vi "Config Spark Max SLOT Close Loop HW Get Set.vi"(4 "PIDF Slot (0)":i32, 6 "Get(f) Set(t)":bool, 7 "SparkMax Slot CL":T1={"Gains"={"P"=0.1, "I"=0.0, "D"=0.0, "F"=0.0}, "I Zone"=1.0, "Peak Out -1 0 1"={"High"=0.0, "Low"=0.0}, "Max I Accu"=0.0} {"Gains"."F" format="%#.8f"; "Gains"."D" format="%#.8f"; "Gains"."I" format="%#.8f"; "Gains"."P" format="%#.8f"; "Peak Out -1 0 1"."Low" format="%#.8f"; "Peak Out -1 0 1"."High" format="%#.8f"}, 8 "Error":errorcluster, 11 "Drive Refs":T4) -> (0 "Error Out":errorcluster, 3 "Drive Refs Out":T4, 5 "SparkMax Slot CL Out":T1={"Gains"={"P"=0.1, "I"=0.0, "D"=0.0, "F"=0.0}, "I Zone"=1.0, "Peak Out -1 0 1"={"High"=0.0, "Low"=0.0}, "Max I Accu"=0.0} {"Gains"."F" format="%#.8f"; "Gains"."D" format="%#.8f"; "Gains"."I" format="%#.8f"; "Gains"."P" format="%#.8f"; "Peak Out -1 0 1"."Low" format="%#.8f"; "Peak Out -1 0 1"."High" format="%#.8f"})   [LabVIEW 2023, in "2024 AdvSwerve_ACT.lvlib"]
uses:
  2024 AdvSwerve_ACT.lvlib
  <vilib>/Rock Robotics/WPI/MotorControl/WPI_MotorControlDeviceRef.ctl
  <vilib>/Rock Robotics/WPI/MotorControl/WPI_MotorControlType.ctl
  <vilib>/Rock Robotics/SystemInterfaces/DIO/FPGA_DIOPWMChannel.ctl
  <vilib>/Rock Robotics/WPI/PWM/WPI_PWMDeadband.ctl
  <vilib>/Rock Robotics/SystemInterfaces/DIO/FPGA_DIOChannel.ctl
  Shared Code/TypeDefs/Cluster_Spark MAX Config_SLOT PID Config.ctl
  Shared Code/TypeDefs/Cluster_PID Gains.ctl
  Shared Code/TypeDefs/Cluster_High-Low.ctl
  Shared Code/TypeDefs/Cluster_SRX SLOT PID Config.ctl
  <vilib>/Utility/error.llb/Trim Whitespace One-Sided.vi
  <vilib>/Utility/Data Type/NI_Data Type.lvlib
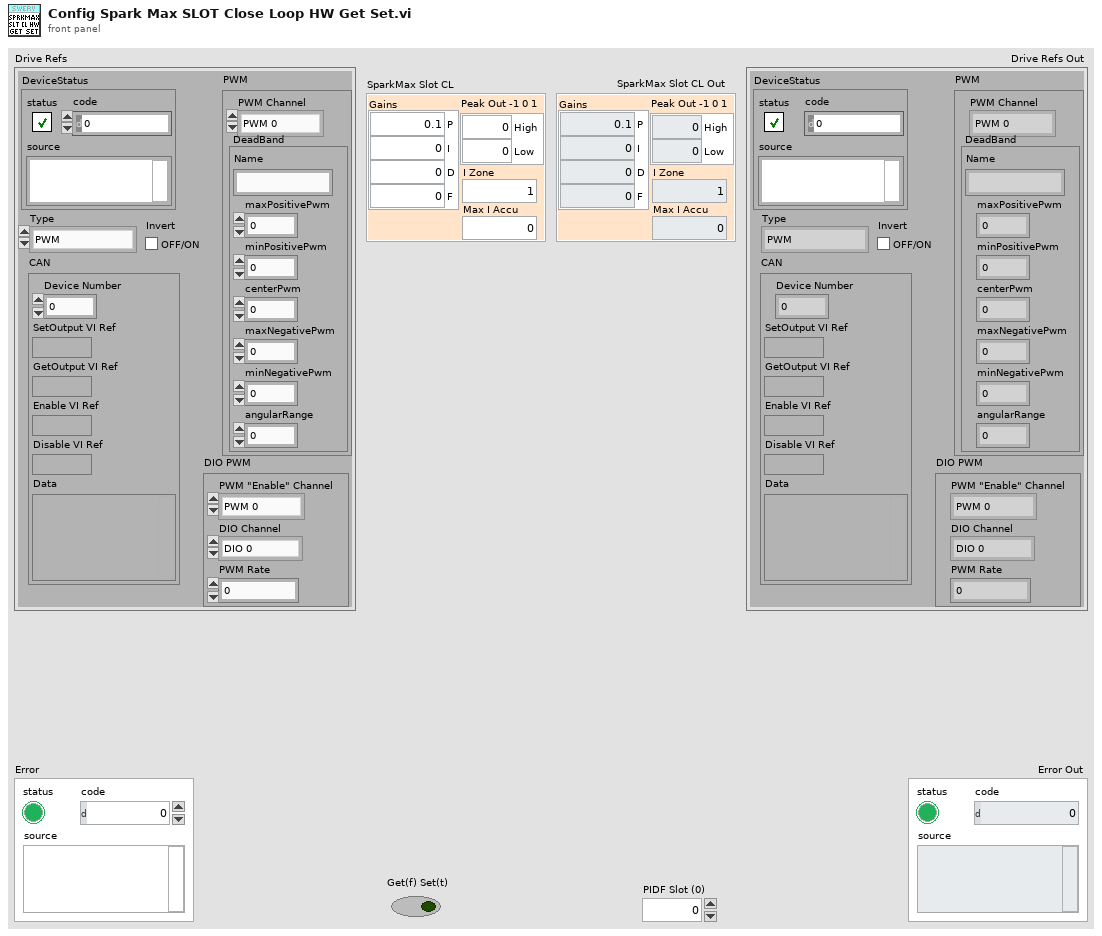
[diagram p1: front panel]
types:
  T1 = typedef "Cluster_Spark MAX Config_SLOT PID Config.ctl" = cluster{"Gains":T2, "I Zone":dbl, "Peak Out -1 0 1":T3, "Max I Accu":dbl}
  T2 = typedef "Cluster_PID Gains.ctl" = cluster{"P":dbl, "I":dbl, "D":dbl, "F":dbl}
  T3 = typedef "Cluster_High-Low.ctl" = cluster{"High":dbl, "Low":dbl}
  T4 = typedef "WPI_MotorControlDeviceRef.ctl" = cluster{"DeviceStatus":errorcluster, "Type":T5, "PWM":cluster{"PWM Channel":T6, "DeadBand":T7}, "CAN":cluster{"Device Number":u8, "SetOutput VI Ref":variant, "GetOutput VI Ref":variant, "Enable VI Ref":variant, "Disable VI Ref":variant, "Data":variant}, "Invert":bool, "DIO PWM":cluster{"PWM \"Enable\" Channel":T6, "DIOChannel":T8, "PWM Rate":dbl}}
  T5 = typedef "WPI_MotorControlType.ctl" = enum16{"PWM", "CAN", "DIO PWM"}
  T6 = typedef "FPGA_DIOPWMChannel.ctl" = enum8{"PWM 0", "PWM 1", "PWM 2", "PWM 3", "PWM 4", "PWM 5", "PWM 6", "PWM 7", "PWM 8", "PWM 9", "PWM MXP 0", "PWM MXP 1", "PWM MXP 2", "PWM MXP 3", "PWM MXP 4", "PWM MXP 5", "PWM MXP 6", "PWM MXP 7", "PWM MXP 8", "PWM MXP 9", "Invalid"}
  T7 = typedef "WPI_PWMDeadband.ctl" = cluster{"Name":string, "maxPositivePwm":i32, "minPositivePwm":i32, "centerPwm":i32, "maxNegativePwm":i32, "minNegativePwm":i32, "angularRange":u16}
  T8 = typedef "FPGA_DIOChannel.ctl" = enum8{"DIO 0", "DIO 1", "DIO 2", "DIO 3", "DIO 4", "DIO 5", "DIO 6", "DIO 7", "DIO 8", "DIO 9", "DIO MXP 0", "DIO MXP 1", "DIO MXP 2", "DIO MXP 3", "DIO MXP 4", "DIO MXP 5", "DIO MXP 6", "DIO MXP 7", "DIO MXP 8", "DIO MXP 9", "DIO MXP 10", "DIO MXP 11", "DIO MXP 12", "DIO MXP 13", "DIO MXP 14", "DIO MXP 15", "SPI Port CS1", "SPI Port CS2", "SPI Port CS3", "SPI Port MISO", "SPI Port MOSI", "Invalid"}
  T9 = typedef "Cluster_SRX SLOT PID Config.ctl" = cluster{"Gains":T2, "Error Allowed":dbl, "I Zone":dbl, "Peak Out 0-1":dbl, "Max I Accu":dbl}
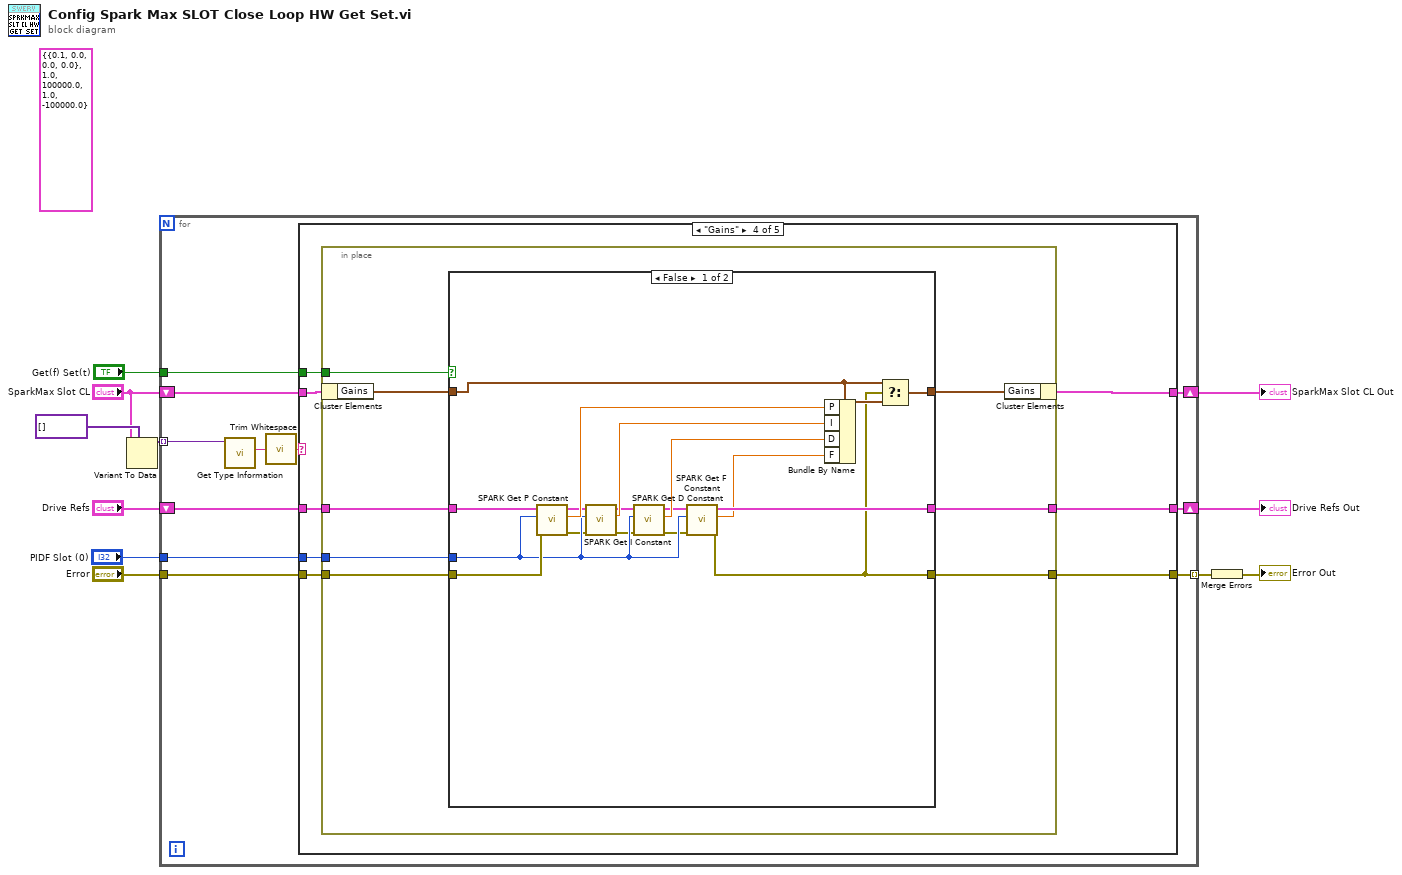
[diagram p0: block diagram]
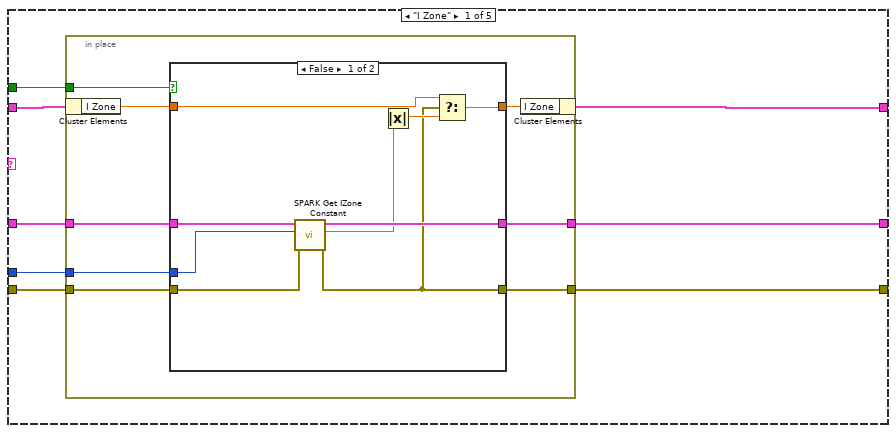
[diagram p2: hidden frame]
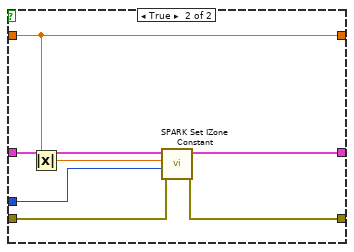
[diagram p3: hidden frame]
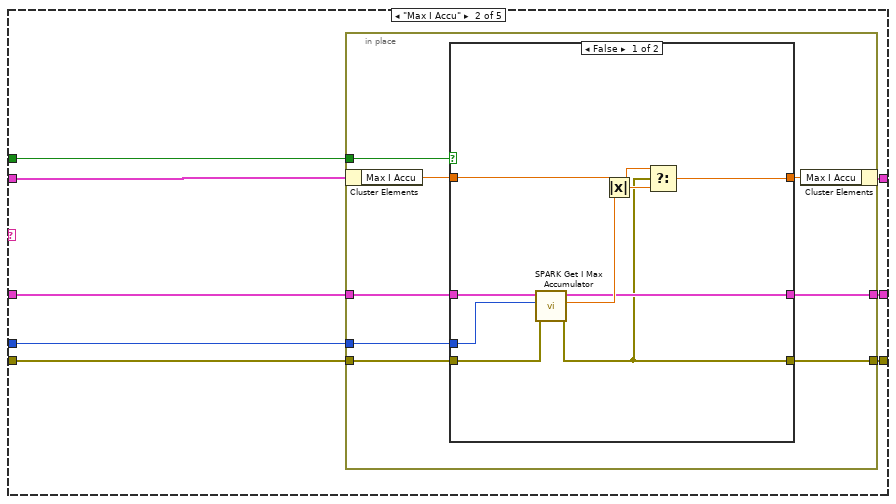
[diagram p4: hidden frame]
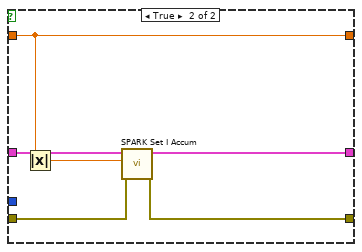
[diagram p5: hidden frame]
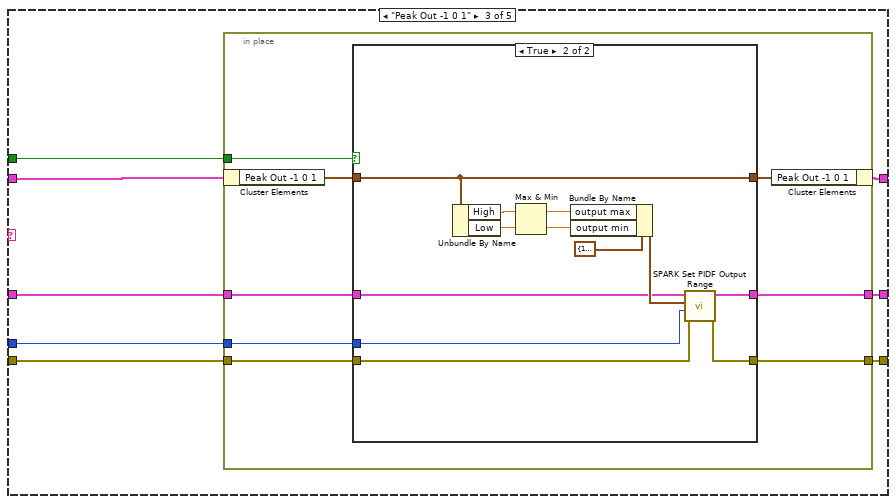
[diagram p6: hidden frame]
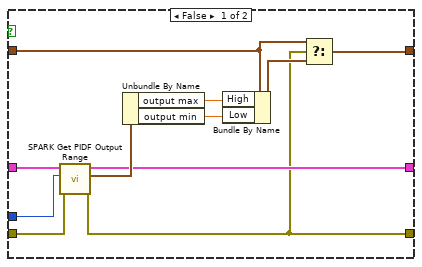
[diagram p7: hidden frame]
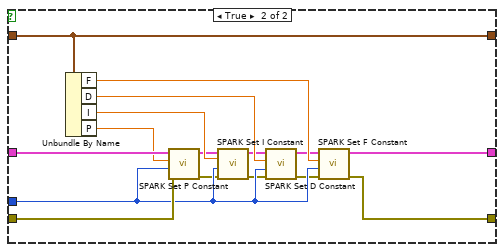
[diagram p8: hidden frame]
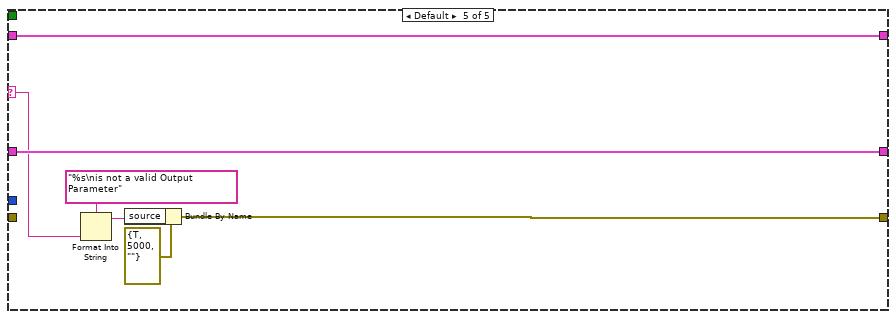
[diagram p9: hidden frame]
diagram:
  (unwired) T9 {"Gains"={"P"=0.1, "I"=0.0, "D"=0.0, "F"=0.0}, "Error Allowed"=1.0, "I Zone"=100000.0, "Peak Out 0-1"=1.0, "Max I Accu"=-100000.0} ("SparkMax Output")
  n1 = Variant To Data(type=variant[] [], Variant="SparkMax Slot CL") -> (data=w6:variant[])  [unwired: 1 in, 1 out]
  n2 = for {
    shift-right: [w13] -> w11
    shift-left: "SparkMax Slot CL" -> [w19]
    shift-right: [w14] -> w9
    shift-left: "Drive Refs" -> [w18]
    tunnel: "Get(f) Set(t)" -> [w17]
    tunnel: w6 -> [w21] mode=indexing
    tunnel: "Error" -> [w16]
    tunnel: [w15] -> w3 mode=indexing
    tunnel: "PIDF Slot (0)" -> [w12]
    n3 = call <vilib>:"Get Type Information.vi"("variant"=w21) -> ("name"=w22:string)  [unwired: 6 in, 4 out]
    n4 = call <vilib>:"Trim Whitespace.vi"("string"=w22) -> ("trimmed string"=w20:string)  [unwired: 1 in]
    n5 = case shown="\"Gains\"" w20 {
      selector: w20 -> [_ _ _ _ w179]
      tunnel: w19 -> [w30 w62 w93 w132 w181]
      tunnel: w18 -> [w26 w58 w89 w128 w180]
      tunnel: w17 -> [w29 w61 w92 w131 _]
      tunnel: w16 -> [w28 w60 w91 w130 _]
      tunnel: [w27 w59 w90 w129 w177] -> w15
      tunnel: [w25 w57 w88 w127 w180] -> w14
      tunnel: [w24 w56 w87 w126 w181] -> w13
      tunnel: w12 -> [w23 w55 w86 w125 _]
      frame "I Zone" {
        n6 = in-place {
          in-place-border: w29 -> [w38]
          in-place-border: w28 -> [w36]
          in-place-border: [w35] -> w27
          in-place-border: w26 -> [w34]
          in-place-border: [w33] -> w25
          in-place-border: w23 -> [w31]
          n7 = in-place-cluster #1(w30) -> ("I Zone"=w37:dbl)
          n8 = case shown="False" w38 {
            tunnel: w37 -> [w46 w54]
            tunnel: w36 -> [w40 w49]
            tunnel: [w39 w48] -> w35
            tunnel: w34 -> [w43 w53]
            tunnel: [w42 w52] -> w33
            tunnel: [w47 w54] -> w32
            tunnel: w31 -> [w44 w50]
            frame False {
              n9 = call <vilib>:"SPARK Get IZone Constant.vi"("error in (no error)"=w40, "PIDF Slot (0)"=w44, "MotorControlDeviceRef in"=w43) -> ("error out"=w39:errorcluster, "IZone"=w41:dbl, "MotorControlDeviceRef out"=w42:T4)  [unwired: 6 in]
              n10 = Absolute Value(x=w41) -> (abs(x)=w45:dbl)
              n11 = Select(t=w46, s=w39, f=w45) -> (s? t:f=w47:dbl)
            }
            frame True {
              n12 = Absolute Value(x=w54) -> (abs(x)=w51:dbl)
              n13 = call <vilib>:"SPARK Set IZone Constant.vi"("error in"=w49, "PIDF Slot"=w50, "IZone"=w51, "MotorControlDeviceRef"=w53) -> ("error out"=w48:errorcluster, "MotorControlDeviceRef"=w52:T4)  [unwired: 6 in]
            }
          }
          n14 = in-place-cluster #1("I Zone"=w32) -> (w24:T1)
        }
      }
      frame "Max I Accu" {
        n15 = in-place {
          in-place-border: w61 -> [w70]
          in-place-border: w60 -> [w68]
          in-place-border: [w67] -> w59
          in-place-border: w58 -> [w66]
          in-place-border: [w65] -> w57
          in-place-border: w55 -> [w63]
          n16 = in-place-cluster #2(w62) -> ("Max I Accu"=w69:dbl)
          n17 = case shown="False" w70 {
            tunnel: w69 -> [w78 w85]
            tunnel: w68 -> [w72 w81]
            tunnel: [w71 w80] -> w67
            tunnel: w66 -> [w74 w84]
            tunnel: [w75 w83] -> w65
            tunnel: [w79 w85] -> w64
            tunnel: w63 -> [w73 _]
            frame False {
              n18 = call <vilib>:"SPARK Get I Max Accumulator.vi"("error in (no error)"=w72, "PIDF Slot (0)"=w73, "MotorControlDeviceRef in"=w74) -> ("error out"=w71:errorcluster, "Max Accumulator"=w76:dbl, "MotorControlDeviceRef out"=w75:T4)  [unwired: 6 in]
              n19 = Absolute Value(x=w76) -> (abs(x)=w77:dbl)
              n20 = Select(t=w78, s=w71, f=w77) -> (s? t:f=w79:dbl)
            }
            frame True {
              n21 = Absolute Value(x=w85) -> (abs(x)=w82:dbl)
              n22 = call <vilib>:"SPARK Set I Accum.vi"("error in"=w81, "I Accum"=w82, "MotorControlDeviceRef"=w84) -> ("error out"=w80:errorcluster, "MotorControlDeviceRef"=w83:T4)  [unwired: 7 in]
            }
          }
          n23 = in-place-cluster #2("Max I Accu"=w64) -> (w56:T1)
        }
      }
      frame "Peak Out -1 0 1" {
        n24 = in-place {
          in-place-border: w92 -> [w101]
          in-place-border: w91 -> [w99]
          in-place-border: [w98] -> w90
          in-place-border: w89 -> [w97]
          in-place-border: [w96] -> w88
          in-place-border: w86 -> [w94]
          n25 = in-place-cluster #3(w93) -> ("Peak Out -1 0 1"=w100:T3)
          n26 = case shown="True" w101 {
            tunnel: w100 -> [w111 w123]
            tunnel: w99 -> [w103 w115]
            tunnel: [w102 w113] -> w98
            tunnel: w97 -> [w105 w117]
            tunnel: [w106 w116] -> w96
            tunnel: [w112 w123] -> w95
            tunnel: w94 -> [w104 w114]
            frame False {
              n27 = call <vilib>:"SPARK Get PIDF Output Range.vi"("error in (no error)"=w103, "PIDF Slot (0)"=w104, "MotorControlDeviceRef in"=w105) -> ("error out"=w102:errorcluster, "output range"=w107:cluster{"output max":dbl, "output min":dbl}, "MotorControlDeviceRef out"=w106:T4)  [unwired: 6 in]
              n28 = Unbundle By Name(w107) -> ("output max"=w109:dbl, "output min"=w108:dbl)
              n29 = Bundle By Name(cluster=w111, "High"=w109, "Low"=w108) -> (w110:T3)
              n30 = Select(t=w111, s=w102, f=w110) -> (s? t:f=w112:T3)
            }
            frame True {
              n31 = Unbundle By Name(w123) -> ("High"=w122:dbl, "Low"=w120:dbl)
              n32 = Max & Min(x=w122, y=w120) -> (max(x,y)=w121:dbl, min(x,y)=w119:dbl)
              n33 = Bundle By Name(cluster=cluster{"output max":dbl, "output min":dbl} {"output max"=1.0, "output min"=-1.0} ("output range"), "output max"=w121, "output min"=w119) -> (w118:cluster{"output max":dbl, "output min":dbl})
              n34 = call <vilib>:"SPARK Set PIDF Output Range.vi"("error in"=w115, "PIDF Slot (0)"=w114, "output range"=w118, "MotorControlDeviceRef"=w117) -> ("error out"=w113:errorcluster, "MotorControlDeviceRef"=w116:T4)  [unwired: 6 in]
            }
          }
          n35 = in-place-cluster #3("Peak Out -1 0 1"=w95) -> (w87:T1)
        }
      }
      frame "Gains" {
        n36 = in-place {
          in-place-border: w131 -> [w140]
          in-place-border: w130 -> [w138]
          in-place-border: [w137] -> w129
          in-place-border: w128 -> [w136]
          in-place-border: [w135] -> w127
          in-place-border: w125 -> [w133]
          n37 = in-place-cluster #4(w132) -> ("Gains"=w139:T2)
          n38 = case shown="False" w140 {
            tunnel: w139 -> [w141 w170]
            tunnel: w138 -> [w153 w171]
            tunnel: [w154 w172] -> w137
            tunnel: w136 -> [w156 w174]
            tunnel: [w155 w173] -> w135
            tunnel: [w158 w170] -> w134
            tunnel: w133 -> [w148 w169]
            frame False {
              n39 = call <vilib>:"SPARK Get P Constant.vi"("error in (no error)"=w153, "PIDF Slot (0)"=w148, "MotorControlDeviceRef in"=w156) -> ("error out"=w144:errorcluster, "kP"=w152:dbl, "MotorControlDeviceRef out"=w147:T4)  [unwired: 6 in]
              n40 = call <vilib>:"SPARK Get I Constant.vi"("error in (no error)"=w144, "PIDF Slot (0)"=w148, "MotorControlDeviceRef in"=w147) -> ("error out"=w143:errorcluster, "kI"=w151:dbl, "MotorControlDeviceRef out"=w146:T4)  [unwired: 6 in]
              n41 = call <vilib>:"SPARK Get D Constant.vi"("error in (no error)"=w143, "PIDF Slot (0)"=w148, "MotorControlDeviceRef in"=w146) -> ("error out"=w142:errorcluster, "kD"=w150:dbl, "MotorControlDeviceRef out"=w145:T4)  [unwired: 6 in]
              n42 = call <vilib>:"SPARK Get F Constant.vi"("error in (no error)"=w142, "PIDF Slot (0)"=w148, "MotorControlDeviceRef in"=w145) -> ("error out"=w154:errorcluster, "kF"=w149:dbl, "MotorControlDeviceRef out"=w155:T4)  [unwired: 6 in]
              n43 = Bundle By Name(cluster=w141, "P"=w152, "I"=w151, "D"=w150, "F"=w149) -> (w157:T2)
              n44 = Select(t=w141, s=w154, f=w157) -> (s? t:f=w158:T2)
            }
            frame True {
              n45 = Unbundle By Name(w170) -> ("F"=w165:dbl, "D"=w166:dbl, "I"=w167:dbl, "P"=w168:dbl)
              n46 = call <vilib>:"SPARK Set P Constant.vi"("error in"=w171, "PIDF Slot"=w169, "kP"=w168, "MotorControlDeviceRef"=w174) -> ("error out"=w161:errorcluster, "MotorControlDeviceRef"=w164:T4)  [unwired: 6 in]
              n47 = call <vilib>:"SPARK Set I Constant.vi"("error in"=w161, "PIDF Slot"=w169, "kI"=w167, "MotorControlDeviceRef"=w164) -> ("error out"=w160:errorcluster, "MotorControlDeviceRef"=w163:T4)  [unwired: 6 in]
              n48 = call <vilib>:"SPARK Set D Constant.vi"("error in"=w160, "PIDF Slot"=w169, "kD"=w166, "MotorControlDeviceRef"=w163) -> ("error out"=w159:errorcluster, "MotorControlDeviceRef"=w162:T4)  [unwired: 6 in]
              n49 = call <vilib>:"SPARK Set F Constant.vi"("error in"=w159, "PIDF Slot"=w169, "kF"=w165, "MotorControlDeviceRef"=w162) -> ("error out"=w172:errorcluster, "MotorControlDeviceRef"=w173:T4)  [unwired: 6 in]
            }
          }
          n50 = in-place-cluster #4("Gains"=w134) -> (w126:T1)
        }
      }
      frame Default {
        n51 = Format Into String(format string="%s\nis not a valid Output Parameter", w179) -> (resulting string=w175:string)  [unwired: 2 in, 1 out]
        n52 = Bundle By Name(cluster=errorcluster {"status"=TRUE, "code"=5000, "source"=""} ("error out"), "source"=w175) -> (w177:errorcluster)
      }
    }
  }
  "Drive Refs Out" <- w9
  "SparkMax Slot CL Out" <- w11
  n53 = Merge Errors(w3) -> (→"Error Out":errorcluster)
